vi "timestring2.vi"(8 "error in (no error)":errorcluster, 10 "String Array In":string[](array[string])) -> (0 "error out":errorcluster, 2 "Time Stamp Out":timestamp[](array[timestamp]) format="%<%X>T")   [LabVIEW 2017]
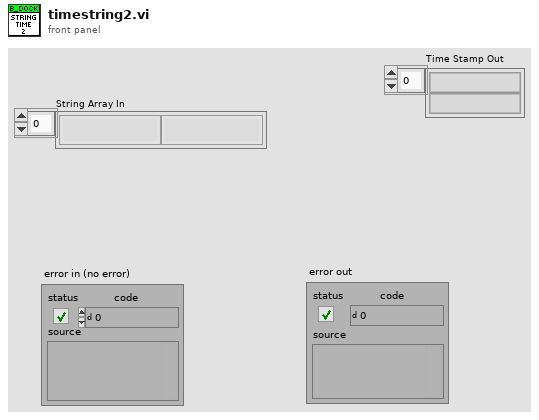
[diagram p1: front panel]
types:
  T1 = cluster{"second":i32, "minute":i32, "hour":i32, "day of month":i32, "month":i32, "year":i32, "day of week":i32, "day of year":i32, "is DST":i32}
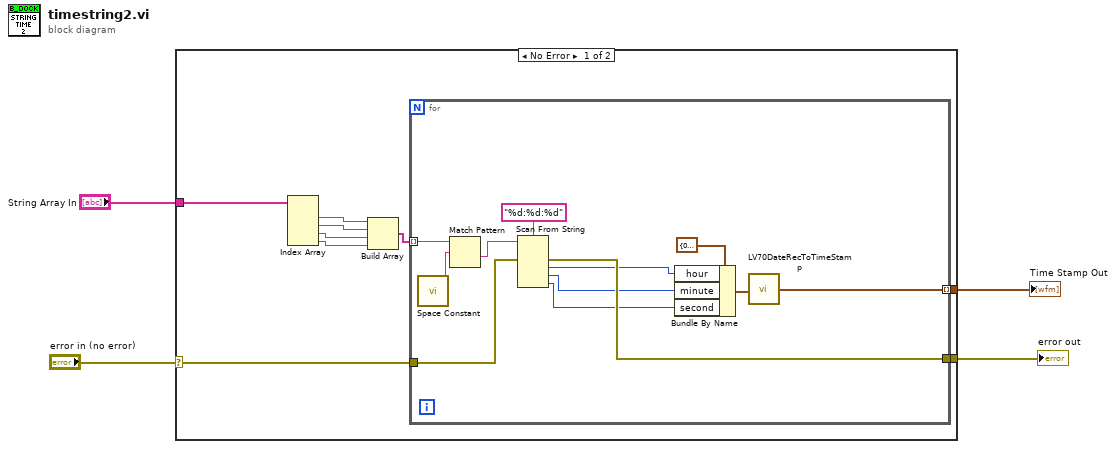
[diagram p0: block diagram]
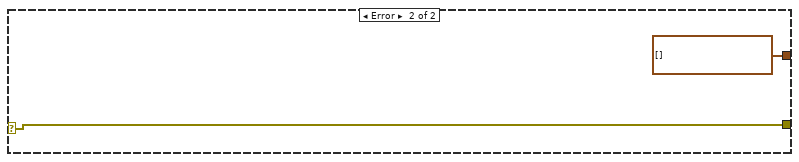
[diagram p2: hidden frame]
diagram:
  n1 = case shown="No Error" "error in (no error)" {
    selector: "error in (no error)" -> [w10 w27]
    tunnel: "String Array In" -> [w13 _]
    tunnel: [w11 timestamp[] []] -> w3
    tunnel: [w9 w27] -> w1
    frame No Error {
      n2 = Index Array(array=w13) -> (element #1=w7:string, element #2=w12:string, element #3=w6:string, element #4=w5:string)  [unwired: 4 in]
      n3 = Build Array(w7, w12, w6, w5) -> (w8:string[])
      n4 = for {
        tunnel: w8 -> [w20] mode=indexing
        tunnel: [w24] -> w11 mode=indexing
        tunnel: w10 -> [w23]
        tunnel: [w22] -> w9
        n5 = call <vilib>:"Space Constant.vi"() -> ("String"=w21:string)
        n6 = Match Pattern(string=w20, regular expression=w21) -> (after substring=w19:string)  [unwired: 1 in, 3 out]
        n7 = Scan From String(format string="%d:%d:%d", input string=w19, error in=w23) -> (error out=w22:errorcluster, output 1=w16:i32, output 2=w15:i32, output 3=w14:i32)  [unwired: 4 in, 2 out]
        n8 = Bundle By Name(cluster=T1 {"second"=0, "minute"=0, "hour"=0, "day of month"=1, "month"=1, "year"=2018, "day of week"=0, "day of year"=0, "is DST"=0} ("date time rec"), "hour"=w16, "minute"=w15, "second"=w14) -> (w18:T1)
        n9 = call <vilib>:"LV70DateRecToTimeStamp.vi"("date time rec"=w18) -> ("Time Stamp"=w24:timestamp)
      }
    }
    frame Error {
    }
  }
  "Time Stamp Out" <- w3
  "error out" <- w1
